vi "Entry.vi"(8 "error in (no error)":errorcluster, 11 "New State":refnum<class "Work.lvclass">) -> (0 "error out":errorcluster, 3 "State out":refnum<class "Work.lvclass">)   [LabVIEW 2024, in "Chef State.lvlib" / "Work.lvclass"]
doc: "This is an abstract method. Override this method to define the behavior when you enter the state."
uses:
  Work.lvclass
  C:/Program Files/National Instruments/LabVIEW 2024/vi.lib/ActorFramework/Actor/Actor.lvclass
  <vilib>/ActorFramework/Actor/Actor.lvclass/Actor.ctl
  Chef UI Logic/Chef UI Logic Messages/Update Log Msg/Update Log Msg.lvclass/Update Log Msg.ctl
  <vilib>/ActorFramework/Message Enqueuer/Message Enqueuer.lvclass/Message Enqueuer.ctl
  <vilib>/ActorFramework/Message Enqueuer/Enqueue.vi
  Chef UI Logic/Chef UI Logic Messages/Update Log Msg/Update Log Msg.lvclass
  C:/Program Files/National Instruments/LabVIEW 2024/vi.lib/ActorFramework/Message/Message.lvclass
  <vilib>/ActorFramework/Message Priority Queue/Priority Enqueue.vi
  Chef State/Chef State.lvclass
  Work.lvclass/Work.ctl
  <vilib>/ActorFramework/Actor/Actor.lvclass
  Worker/Worker Messages/Test Methods Msg/Test Methods Msg.lvclass
  C:/Users/burakkorkmaz/Desktop/PROJE/actor-state-machine/Chef State/Chef State/Chef State.lvclass
  C:/Program Files/National Instruments/LabVIEW 2024/vi.lib/NI/Actors/State Actor/State Actor/State Actor.lvclass
  C:/Users/burakkorkmaz/Desktop/PROJE/actor-state-machine/Chef State/Work/Work.lvclass
  C:/Users/burakkorkmaz/Desktop/PROJE/actor-state-machine/Chef State Logic/Work Logic/Work Logic.lvclass
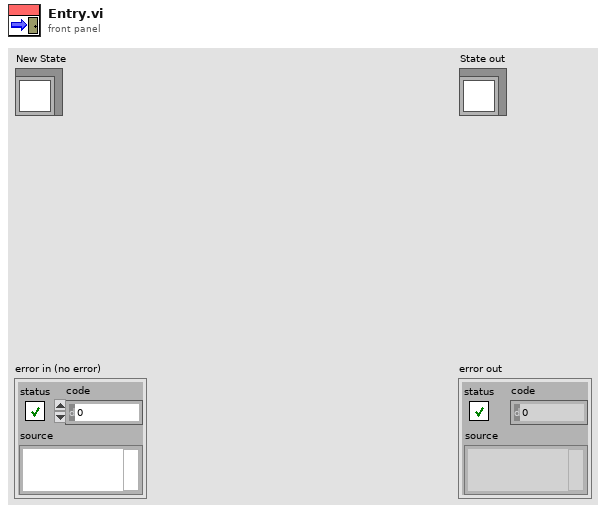
[diagram p1: front panel]
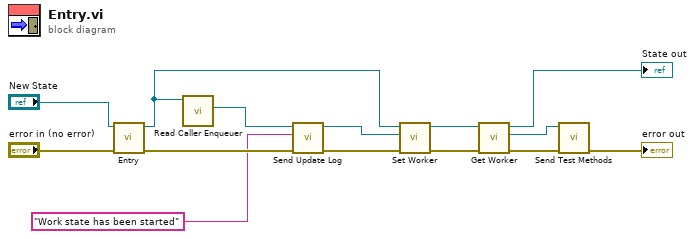
[diagram p0: block diagram]
diagram:
  n1 = call-parent "Entry.vi"("error in (no error)"="error in (no error)", "New State"="New State") -> ("error out"=w11:errorcluster, "State out"=w6:refnum<class "Work.lvclass">)  [unwired: 8 in]
  n2 = call <vilib>:"Read Caller Enqueuer.vi"("Actor"=w6) -> ("Caller Enqueuer"=w12:refnum<class "Message Enqueuer.lvclass">)  [unwired: 10 in]
  n3 = call "Send Update Log.vi"("error in (no error)"=w11, "Log"="Work state has been started", "Message Enqueuer"=w12) -> ("error out"=w8:errorcluster, "Message Enqueuer out"=w9:refnum<class "Message Enqueuer.lvclass">)  [unwired: 7 in]
  n4 = call-dynamic "Set Worker.vi"("error in (no error)"=w8, "Worker"=w9, "Chef State in"=w6) -> ("error out"=w7:errorcluster, "Chef State out"=w3:refnum<class "Work.lvclass">)  [unwired: 7 in]
  n5 = call-dynamic "Get Worker.vi"("error in (no error)"=w7, "Chef State in"=w3) -> ("error out"=w4:errorcluster, "Worker"=w1:refnum<class "Message Enqueuer.lvclass">, "Chef State out"=→"State out":refnum<class "Work.lvclass">)  [unwired: 7 in]
  n6 = call "Send Test Methods.vi"("error in (no error)"=w4, "Message Enqueuer"=w1) -> ("error out"=→"error out":errorcluster)  [unwired: 8 in, 1 out]
